vi "Create Surface.vi"(6 "Draw Mode":T8(ring)=enum."Triangles", 7 "3D Contour Property":T4={"General Property"={"Plot Name"="", "Coordinate System"=enum."Cartesian", "Opacity"=0.0}, "Projection Property"={"Draw XY"=FALSE, "Draw YZ"=FALSE, "Draw XZ"=FALSE}, "Plot Property"={"Line Style"=enum."None", "Line Width"=2.0, "Line Color"=0, "Antialiasing"=FALSE, "Color Ramp Cluster"={"Color Ramp Style"=enum."None", "Color Ramp Array"=[16711934, 393471, 57855, 4390754, 16449346, 16744722, 16711680], "Color Ramp Index"=[45, 91, 133, 175, 219, 255], "Interpolate?"=FALSE, "Logarithm?"=FALSE}}, "Contour Property"={"Contour Type"=enum."Contour", "Axis Basis"=enum."Z-Axis", "Level List"=[], "Level Mode"=enum."Levels", "Levels"=0, "Interval"=0.0}}, 8 "error in (no error)":errorcluster, 9 "Actual Transform In":T7, 10 "Plot Representation In":T1, 11 "Plot Object In":refnum<vi>) -> (0 "error out":errorcluster, 1 "Actual Transform Out":T7, 2 "Plot Representation Out":T1, 3 "Plot Object Out":refnum<vi>, 4 "Surface Object Out":refnum<vi>)   [LabVIEW 2017, in "3D Contour.lvclass"]
uses:
  <vilib>/Math Plots/3D Math Plots/3D Contour/3D Contour/3D Contour.lvclass
  <vilib>/Math Plots/3D Math Plots/3D Plot/3D Plot/Typedef/Actual Transform.ctl
  <vilib>/Math Plots/3D Math Plots/3D Plot/3D Plot/Typedef/Range Clusters.ctl
  <vilib>/Math Plots/3D Math Plots/3D Contour/3D Contour/Typedef/3D Contour Property.ctl
  <vilib>/Math Plots/3D Math Plots/3D Plot/3D Plot/Typedef/Line Type.ctl
  <vilib>/Math Plots/3D Math Plots/3D Plot/3D Plot/Typedef/Color Ramp Cluster.ctl
  <vilib>/Math Plots/3D Math Plots/3D Plot/3D Plot/Typedef/Plot Representation.ctl
  <vilib>/Math Plots/3D Math Plots/3D Plot/3D Plot/Typedef/Mesh Data.ctl
  <vilib>/picture/3D Picture Control/NI_3D Picture Control.lvlib
  <vilib>/Math Plots/3D Math Plots/3D Plot/3D Plot/3D Plot.lvclass
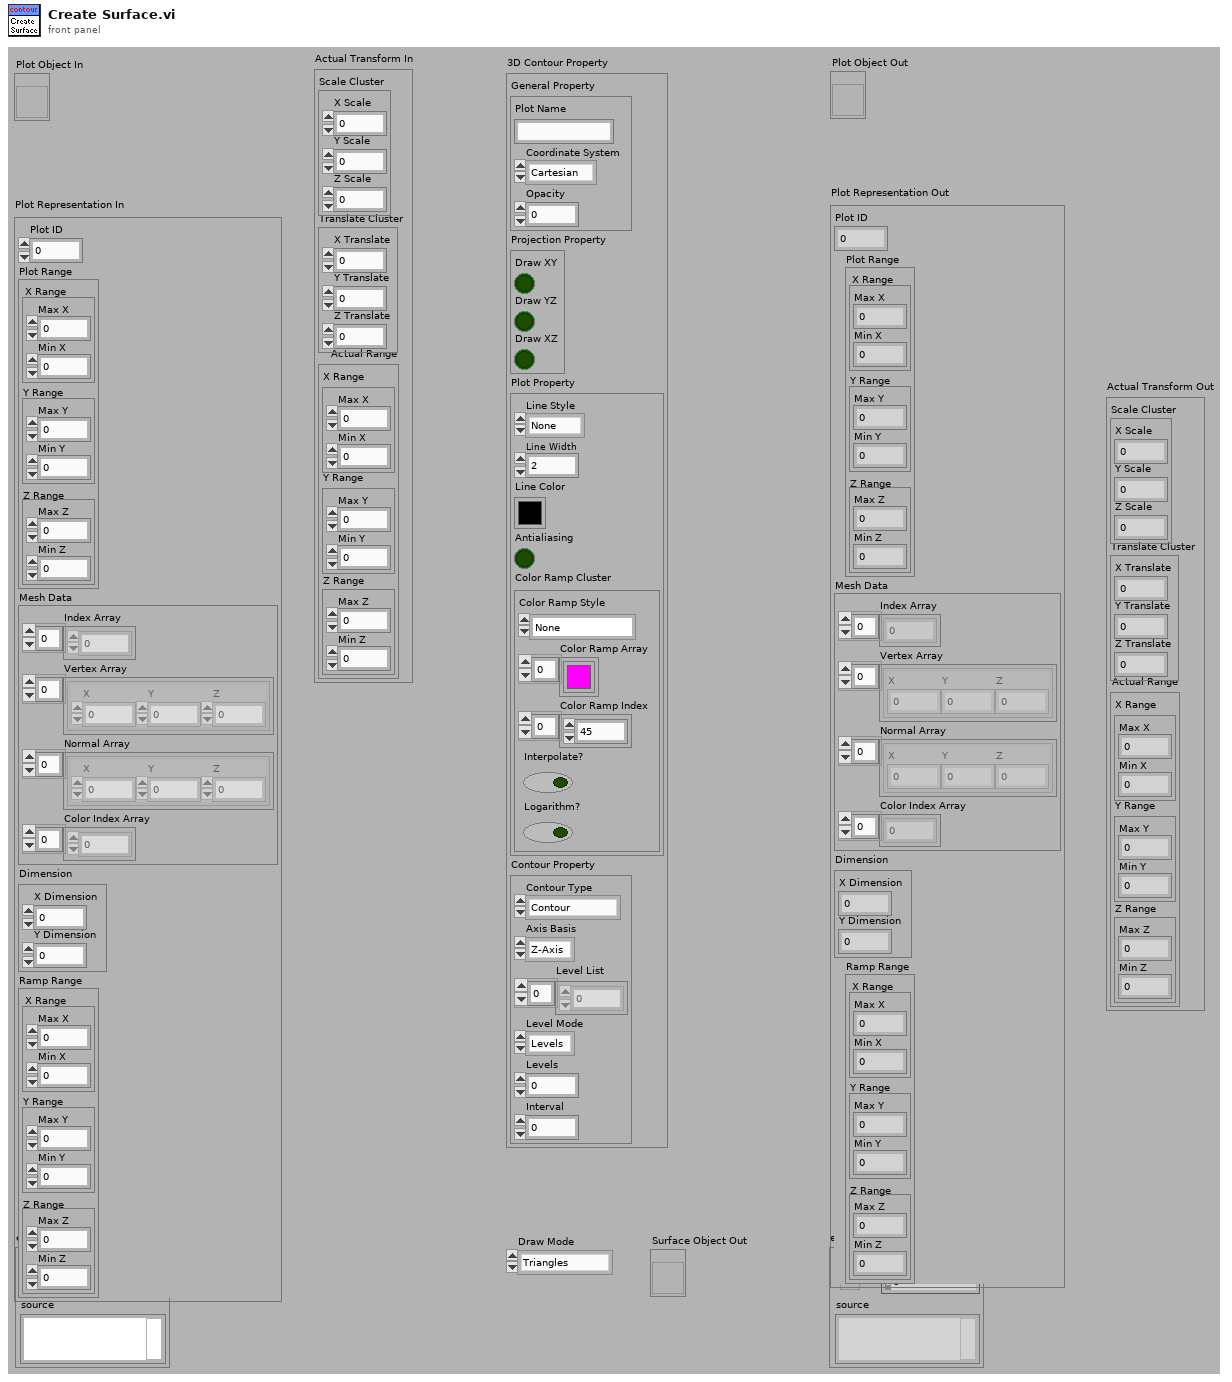
[diagram p1: front panel]
types:
  T1 = typedef "3D Plot.lvclass/Plot Representation.ctl" = cluster{"Plot ID":i32, "Plot Range":T2, "Mesh Data":T3, "Dimension":cluster{"X Dimension":i32, "Y Dimension":i32}, "Ramp Range":T2}
  T2 = typedef "3D Plot.lvclass/Range Clusters.ctl" = cluster{"X Range":cluster{"Max X":sgl, "Min X":sgl}, "Y Range":cluster{"Max Y":sgl, "Min Y":sgl}, "Z Range":cluster{"Max Z":sgl, "Min Z":sgl}}
  T3 = typedef "3D Plot.lvclass/Mesh Data.ctl" = cluster{"Index Array":u32[], "Vertex Array":cluster{"X":sgl, "Y":sgl, "Z":sgl}[], "Normal Array":cluster{"X":sgl, "Y":sgl, "Z":sgl}[], "Color Index Array":i32[]}
  T4 = typedef "3D Contour.lvclass/3D Contour Property.ctl" = cluster{"General Property":cluster{"Plot Name":string, "Coordinate System":enum16{"Cartesian", "Cylindrical", "Spherical"}, "Opacity":sgl}, "Projection Property":cluster{"Draw XY":bool, "Draw YZ":bool, "Draw XZ":bool}, "Plot Property":cluster{"Line Style":T5, "Line Width":sgl, "Line Color":u32, "Antialiasing":bool, "Color Ramp Cluster":T6}, "Contour Property":cluster{"Contour Type":enum16{"Contour", "Contour with surface"}, "Axis Basis":enum16{"X-Axis", "Y-Axis", "Z-Axis"}, "Level List":sgl[], "Level Mode":enum16{"Levels", "Interval", "Level List"}, "Levels":u16, "Interval":sgl}}
  T5 = typedef "3D Plot.lvclass/Line Type.ctl" = enum16{"None", "Solid", "Dash", "Dot", "Dash Dot"}
  T6 = typedef "3D Plot.lvclass/Color Ramp Cluster.ctl" = cluster{"Color Ramp Style":enum16{"None", "Shaded", "Color spectrum", "Grey scale", "Custom"}, "Color Ramp Array":u32[], "Color Ramp Index":i32[], "Interpolate?":bool, "Logarithm?":bool}
  T7 = typedef "3D Plot.lvclass/Actual Transform.ctl" = cluster{"Scale Cluster":cluster{"X Scale":sgl, "Y Scale":sgl, "Z Scale":sgl}, "Translate Cluster":cluster{"X Translate":sgl, "Y Translate":sgl, "Z Translate":sgl}, "Actual Range":T2}
  T8 = enum16{"Points", "Lines", "Line Strip", "Line Loop", "Triangles", "Triangle Strip", "Triangle Fan", "Quads", "Quad Strip", "Polygon"}
  T9 = enum16{"Overall", "Per Primitive", "Per Vertex", "Binding Off"}
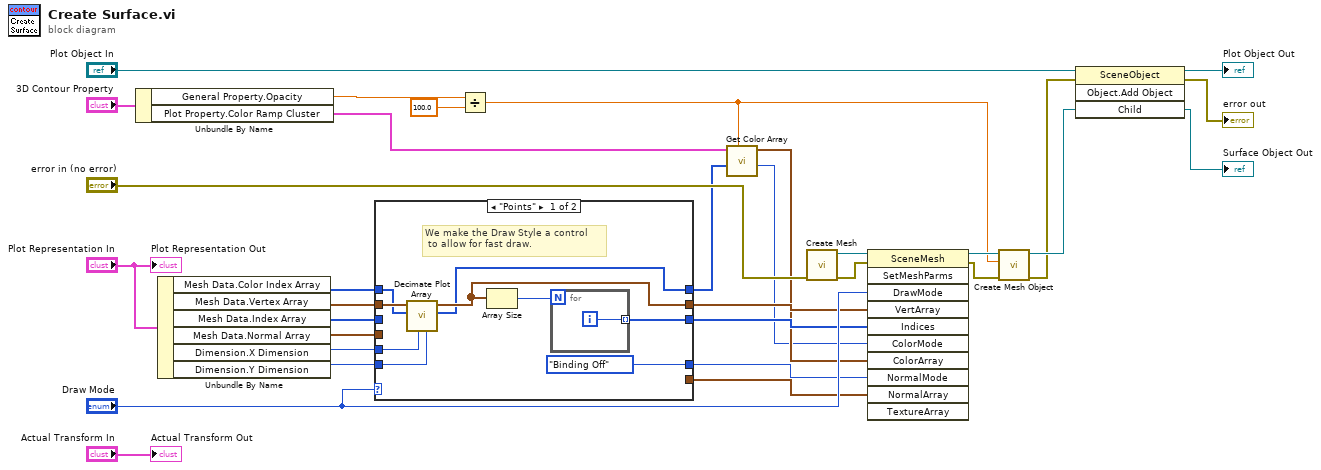
[diagram p0: block diagram]
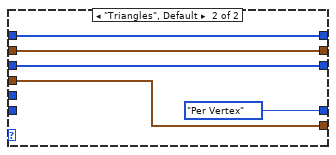
[diagram p2: hidden frame]
diagram:
  n1 = Unbundle By Name("3D Contour Property") -> ("General Property.Opacity"=w24:sgl, "Plot Property.Color Ramp Cluster"=w2:T6)
  n2 = Unbundle By Name("Plot Representation In") -> ("Mesh Data.Color Index Array"=w5:i32[], "Mesh Data.Vertex Array"=w21:cluster{"X":sgl, "Y":sgl, "Z":sgl}[], "Mesh Data.Index Array"=w20:u32[], "Mesh Data.Normal Array"=w18:cluster{"X":sgl, "Y":sgl, "Z":sgl}[], "Dimension.X Dimension"=w12:i32, "Dimension.Y Dimension"=w11:i32)
  n3 = case shown="\"Points\"" "Draw Mode" {
    tunnel: w21 -> [w40 w46]
    tunnel: [w37 w46] -> w15
    tunnel: w20 -> [_ w45]
    tunnel: [w34 w45] -> w19
    tunnel: w18 -> [_ w47]
    tunnel: [_ w47] -> w17
    tunnel: w12 -> [w39 _]
    tunnel: w11 -> [w38 _]
    tunnel: w5 -> [w36 w44]
    tunnel: [w35 w44] -> w4
    tunnel: [T9."Binding Off" ("Normal Binding Mode") T9."Per Vertex" ("Normal Binding Mode")] -> w1
    frame "Points" {
      # "We make the Draw Style a control\n to allow for fast draw."
      n4 = call <vilib>:"Decimate Plot Array.vi"("Y Dimension"=w38, "X Dimension"=w39, "Color Index Array In"=w36, "Vertex Array In"=w40) -> ("Color Index Array Out"=w35:i32[], "Vertex Array Out"=w37:cluster{"X":sgl, "Y":sgl, "Z":sgl}[])  [unwired: 1 in, 5 out]
      n5 = Array Size(array=w37) -> (size(s)=w41:i32)
      n6 = for {
        N: w41 -> [_]
        tunnel: [w42] -> w34 mode=indexing
        i -> [w42]
      }
    }
    frame "Triangles", Default {
    }
  }
  n7 = Divide(x=w24, y=sgl 100.0) -> (x/y=w3:sgl)
  n8 = call <vilib>:"Get Color Array.vi"("Alpha"=w3, "Color Index Array"=w4, "Color Ramp Cluster"=w2) -> ("Color Binding Mode"=w13:T9, "Color Array"=w14:cluster{"R":sgl, "G":sgl, "B":sgl, "A":sgl}[])  [unwired: 4 in, 3 out]
  n9 = call <vilib>:"Create Mesh.vi"("error in (no error)"="error in (no error)") -> ("error out"=w16:errorcluster, "New Mesh Refnum"=w23:refnum<vi>)  [unwired: 9 out]
  n10 = invoke class="SceneMesh" method="SetMeshParms"(reference=w23, error in=w16, "DrawMode"="Draw Mode", "VertArray"=w15, "Indices"=w19, "ColorMode"=w13, "ColorArray"=w14, "NormalMode"=w1, "NormalArray"=w17) -> (reference out=w10:refnum<vi>, error out=w9:errorcluster)  [unwired: 2 in, 9 out]
  n11 = call <vilib>:"Create Mesh Object.vi"("error in (no error)"=w9, "Alpha"=w3, "Mesh Object In"=w10) -> ("error out"=w7:errorcluster, "Object Ref Out"=w8:refnum<vi>)  [unwired: 1 in, 6 out]
  n12 = invoke class="SceneObject" method="Object.Add Object"(reference="Plot Object In", error in=w7, "Child"=w8) -> (reference out=→"Plot Object Out":refnum<vi>, error out=→"error out":errorcluster, "Child"=→"Surface Object Out":refnum<vi>)  [unwired: 1 in, 1 out]
  "Actual Transform Out" <- "Actual Transform In"
  "Plot Representation Out" <- "Plot Representation In"
